vi "InterpretStructure.vi"(5 "Structure in":refnum<class "Structure.lvclass">, 6 "error in":errorcluster, 9 "VI Interpreter in":refnum<class "VI Interpreter.lvclass">) -> (0 "error out":errorcluster, 3 "VI Interpreter out":refnum<class "VI Interpreter.lvclass">, 4 "Structure out":refnum<class "Structure.lvclass">)   [LabVIEW 2014, in "Raspberry Pi Compatible Compiler for LabVIEW.lvlib" / "VI Interpreter.lvclass"]
uses:
  VI Interpreter.lvclass
  Structure/Structure.lvclass
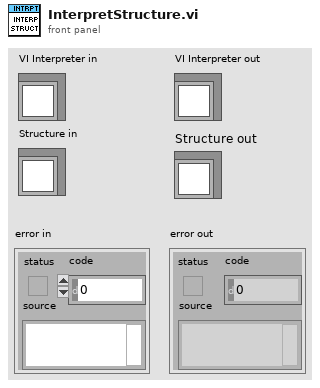
[diagram p1: front panel]
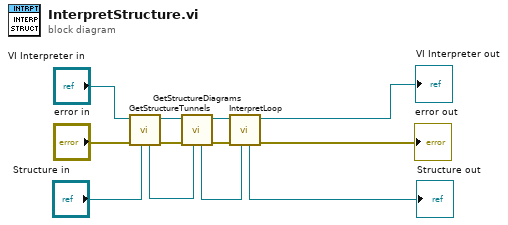
[diagram p0: block diagram]
diagram:
  n1 = call "GetStructureTunnels.vi"("Structure in"="Structure in", "error in"="error in", "VI Interpreter in"="VI Interpreter in") -> ("error out"=w9:errorcluster, "VI Interpreter out"=w8:refnum<class "VI Interpreter.lvclass">, "Structure out"=w7:refnum<class "Structure.lvclass">)  [unwired: 4 in]
  n2 = call "GetStructureDiagrams.vi"("Structure in"=w7, "error in"=w9, "VI Interpreter in"=w8) -> ("error out"=w5:errorcluster, "VI Interpreter out"=w6:refnum<class "VI Interpreter.lvclass">, "Structure out"=w4:refnum<class "Structure.lvclass">)  [unwired: 4 in]
  n3 = call "InterpretLoop.vi"("Structure in"=w4, "error in"=w5, "VI Interpreter in"=w6) -> ("error out"=→"error out":errorcluster, "VI Interpreter out"=→"VI Interpreter out":refnum<class "VI Interpreter.lvclass">, "Structure out"=→"Structure out":refnum<class "Structure.lvclass">)  [unwired: 4 in]
